vi "Graph AddCursor(XY).vi"(8 "エラー入力（エラーなし）":errorcluster, 9 "色":u32(colorbox), 10 "名称":string, 11 "XYグラフref":refnum<vi>) -> (0 "エラー出力":errorcluster)   [LabVIEW 2014]
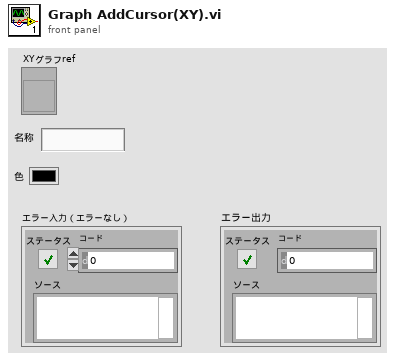
[diagram p1: front panel]
types:
  T1 = cluster{"Name":string, "Color":u32, "Style":u8, "Point Style":u8, "Name Visible":bool, "Allow Drag":bool, "Cursor Mode":u32, "Plot":i32, "Index":i32, "Position":cluster{"X":dbl, "Y":dbl}, "X Scale":u32, "Y Scale":u32, "Watch Plots":i32[], "Watch All Plots":bool, "Plot Area":i32, "Label Offset":cluster{"X":dbl, "Y":dbl}}
  T2 = typedef "LVCursorListTypeDef.ctl" = cluster{"Name":string, "Color":u32, "Style":u8, "Point Style":u8, "Name Visible":bool, "Allow Drag":bool, "Cursor Mode":u32, "Plot":i32, "Index":i32, "Position":cluster{"X":dbl, "Y":dbl}, "X Scale":u32, "Y Scale":u32, "Watch Plots":i32[], "Watch All Plots":bool, "Plot Area":i32, "Label Offset":cluster{"X":dbl, "Y":dbl}}[]
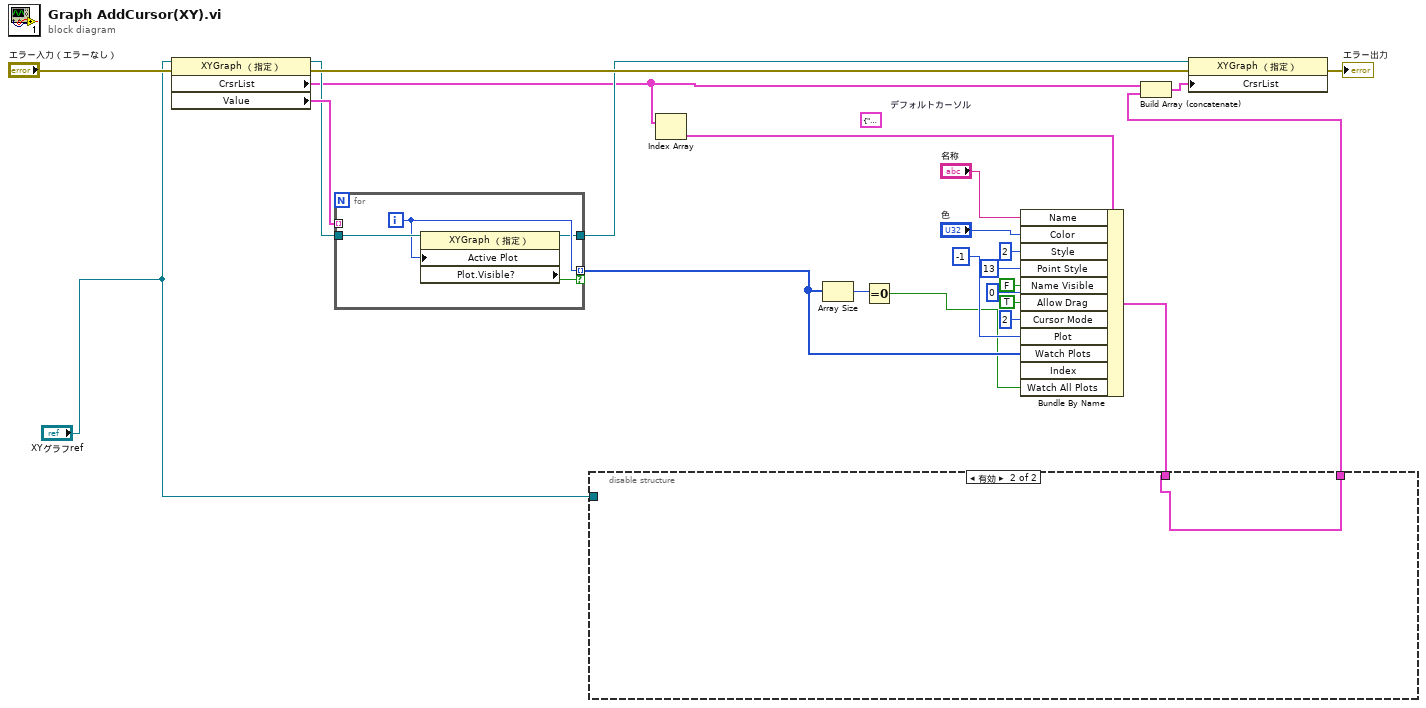
[diagram p0: block diagram]
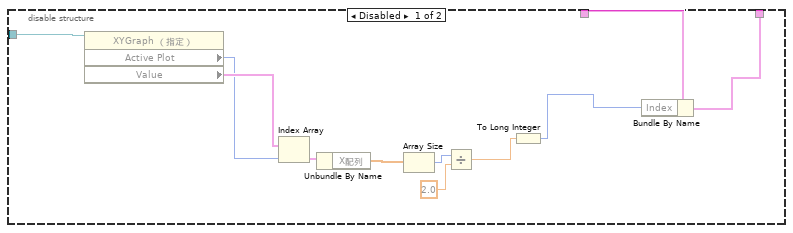
[diagram p2: hidden frame]
diagram:
  (unwired) T1 {"Name"="カーソル0", "Color"=16776960, "Style"=2, "Point Style"=13, "Name Visible"=FALSE, "Allow Drag"=TRUE, "Cursor Mode"=2, "Plot"=-1, "Index"=42, "Position"={"X"=0.42, "Y"=43.0}, "X Scale"=0, "Y Scale"=0, "Watch Plots"=[], "Watch All Plots"=TRUE, "Plot Area"=0, "Label Offset"={"X"=-0.0012080536912751905, "Y"=172.10516252390056}}  # デフォルトカーソル
  n1 = property class="XYGraph （指定）"(reference="XYグラフref", error in="エラー入力（エラーなし）") -> (reference out=w12:refnum<vi>, error out=w18:errorcluster, "CrsrList"=w2:T2, "Value"=w23:cluster{"X配列":dbl[], "Y配列":dbl[]}[])
  n2 = for {
    tunnel: w12 -> [w28]
    tunnel: w23 -> [_] mode=indexing
    tunnel: [w27] -> w11 mode=indexing if=w26
    tunnel: [w25] -> w13
    i -> [w27]
    n3 = property class="XYGraph （指定）"(reference=w28, "Active Plot"=w27) -> (reference out=w25:refnum<vi>, "Plot.Visible?"=w26:bool)  [unwired: 1 in, 1 out]
  }
  n4 = Index Array(array=w2) -> (element=w1:T1)  [unwired: 1 in]
  n5 = Array Size(array=w11) -> (size(s)=w10:i32)
  n6 = Equal To 0?(x=w10) -> (x = 0?=w9:bool)
  n7 = Bundle By Name(cluster=w1, "Name"="名称", "Color"="色", "Style"=u8 2, "Point Style"=u8 13, "Name Visible"=FALSE, "Allow Drag"=TRUE, "Cursor Mode"=u32 2, "Plot"=-1, "Watch Plots"=w11, "Index"=0, "Watch All Plots"=w9) -> (w15:T1)
  n8 = disable-structure shown="有効" {
    disable-tunnel: w15 -> [w39 w40]
    disable-tunnel: [w38 w40] -> w14
    disable-tunnel: "XYグラフref" -> [w37 _]
    frame Disabled {
      n9 = property class="XYGraph （指定）"(reference=w37) -> ("Active Plot"=w35:u32, "Value"=w36:cluster{"X配列":dbl[], "Y配列":dbl[]}[])  [unwired: 1 in, 2 out]
      n10 = Index Array(array=w36, index=w35) -> (element=w33:cluster{"X配列":dbl[], "Y配列":dbl[]})
      n11 = Unbundle By Name(w33) -> ("X配列"=w32:dbl[])
      n12 = Array Size(array=w32) -> (size(s)=w31:i32)
      n13 = Divide(x=w31, y=2.0) -> (x/y=w29:dbl)
      n14 = To Long Integer(number=w29) -> (32bit integer=w34:i32)
      n15 = Bundle By Name(cluster=w39, "Index"=w34) -> (w38:T1)
    }
    frame Enabled {
    }
  }
  n16 = Build Array (concatenate)(w2, w14) -> (w20:T2)
  n17 = property class="XYGraph （指定）"(reference=w13, error in=w18, "CrsrList"=w20) -> (error out=→"エラー出力":errorcluster)  [unwired: 1 out]
